vi "GetMatlabTempParamData.vi"(10 "index":dbl, 11 "ExpID":string) -> (3 "Matlab param data":T1[](array[typedef]))   [LabVIEW 2017]
uses:
  Types/MatlabDataBundle.ctl
  Types/MatlabDataType.ctl
panel:
  out "Param Data before convert":T1[](array[typedef])
  in  "Clear Temp?":bool=TRUE
  out "error out":errorcluster
  in  "error in":errorcluster
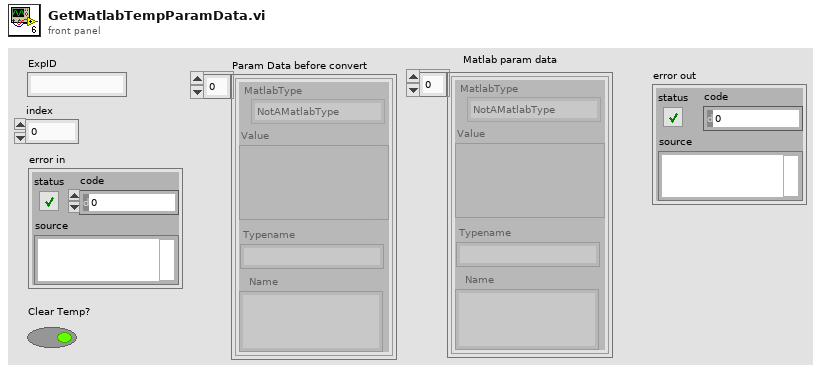
[diagram p1: front panel]
types:
  T1 = typedef "MatlabDataBundle.ctl" = cluster{"MatlabType":T2, "Value":variant, "Name":string, "Typename":string}
  T2 = typedef "MatlabDataType.ctl" = enum16{"NotAMatlabType", "Real", "Complex", "String", "Boolean"}
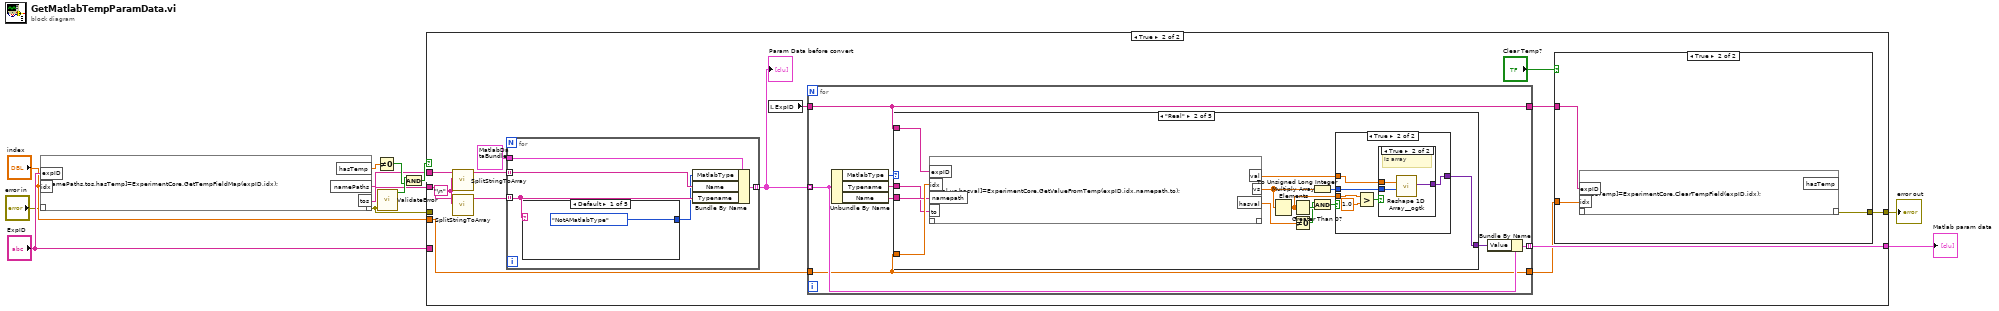
[diagram p0: block diagram]
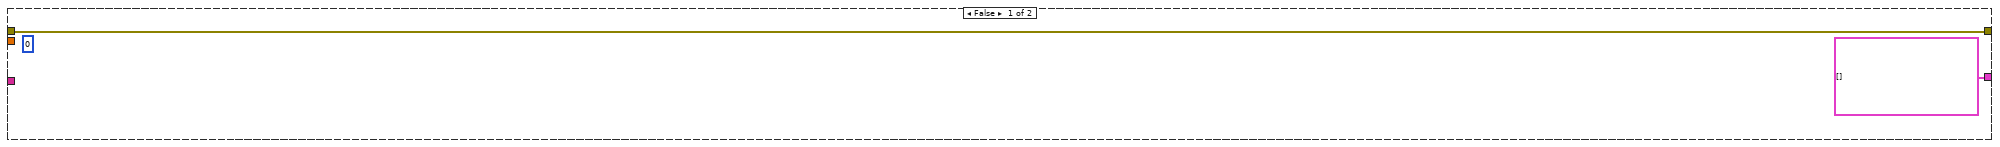
[diagram p2: hidden frame]
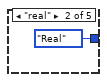
[diagram p3: hidden frame]
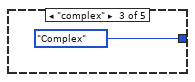
[diagram p4: hidden frame]
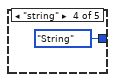
[diagram p5: hidden frame]
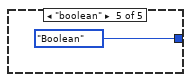
[diagram p6: hidden frame]
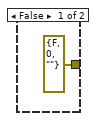
[diagram p7: hidden frame]
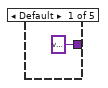
[diagram p8: hidden frame]
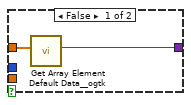
[diagram p9: hidden frame]
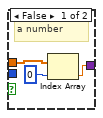
[diagram p10: hidden frame]
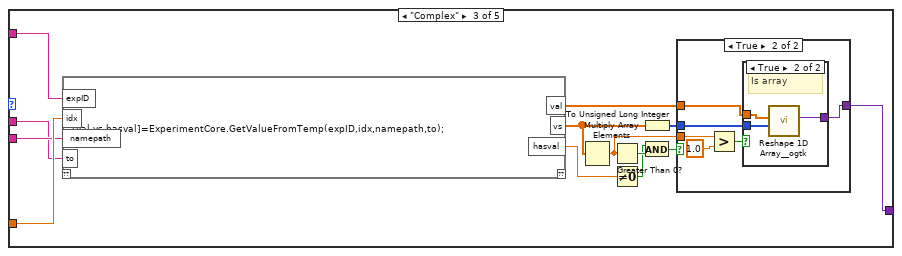
[diagram p11: hidden frame]
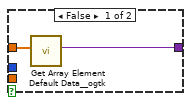
[diagram p12: hidden frame]
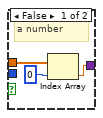
[diagram p13: hidden frame]
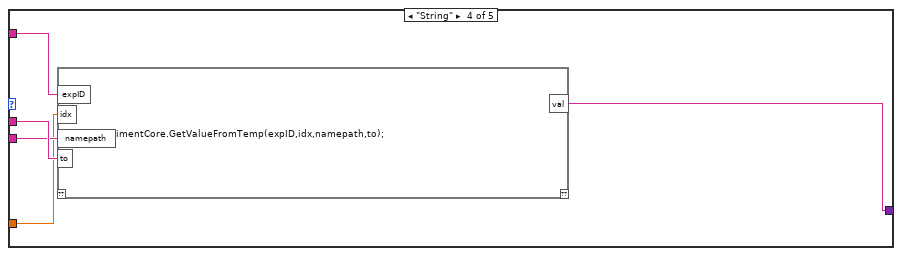
[diagram p14: hidden frame]
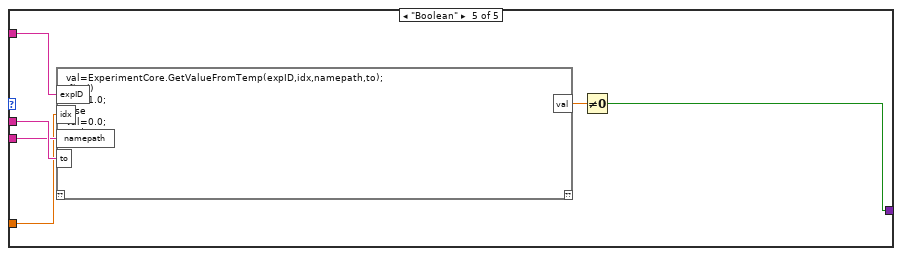
[diagram p15: hidden frame]
diagram:
  n1 = script code="[namePaths,tos,hasTemp]=ExperimentCore.GetTempFieldMap(expID,idx);"("??"="error in", "expID"="ExpID", "idx"="index") -> ("??"=w8:errorcluster, "hasTemp"=w11:dbl, "namePaths"=w1:string, "tos"=w2:string)
  n2 = Not Equal To 0?(x=w11) -> (x != 0?=w6:bool)
  n3 = call "ValidateError.vi"("error in (no error)"=w8) -> ("NoError?"=w7:bool)  [unwired: 9 in, 1 out]
  n4 = And(x=w7, y=w6) -> (x .and. y?=w5:bool)
  n5 = case shown="True" w5 {
    tunnel: [T1[] [] w28] -> w12
    tunnel: "ExpID" -> [_ _]
    tunnel: "index" -> [_ w27]
    tunnel: w8 -> [w13 _]
    tunnel: [w13 w16] -> w3
    tunnel: w2 -> [_ w21]
    tunnel: w1 -> [_ w20]
    frame False {
      (unwired) 0
    }
    frame True {
      w22 = "\n"
      n6 = call "SplitStringToArray.vi"("search string/char (-)"=w22, "String in"=w20) -> ("Split(s)"=w24:string[])  [unwired: 9 in]
      n7 = call "SplitStringToArray.vi"("search string/char (-)"=w22, "String in"=w21) -> ("Split(s)"=w25:string[])  [unwired: 9 in]
      n8 = for {
        tunnel: w24 -> [w32] mode=indexing
        tunnel: w25 -> [w30] mode=indexing
        tunnel: T1 {"MatlabType"=enum."NotAMatlabType", "Value"=variant, "Name"="", "Typename"=""} ("MatlabDataBundle") -> [w33]
        tunnel: [w31] -> w19 mode=indexing
        n9 = case shown="Default" w30 {
          tunnel: [MatlabDataType."NotAMatlabType" ("MatlabType") MatlabDataType."Real" ("MatlabType") MatlabDataType."Complex" ("MatlabType") MatlabDataType."String" ("MatlabType") MatlabDataType."Boolean" ("MatlabType")] -> w29
          frame Default {
          }
          frame "real" {
          }
          frame "complex" {
          }
          frame "string" {
          }
          frame "boolean" {
          }
        }
        n10 = Bundle By Name(cluster=w33, "MatlabType"=w29, "Name"=w32, "Typename"=w30) -> (w31:T1)
      }
      "Param Data before convert" <- w19
      n11 = local read "ExpID"() -> (w18:string)
      n12 = for {
        tunnel: w19 -> [w47] mode=indexing
        tunnel: [w46] -> w28 mode=indexing
        tunnel: w27 -> [w43]
        tunnel: w18 -> [w44]
        tunnel: [w44] -> w17
        tunnel: [w43] -> w15
        n13 = Unbundle By Name(w47) -> ("MatlabType"=w45:T2, "Typename"=w50:string, "Name"=w49:string)
        n14 = case shown="\"Real\"" w45 {
          tunnel: [variant ("Reshaped VArray") w58 w85 w110 w115] -> w48
          tunnel: w44 -> [_ w64 w91 w109 w114]
          tunnel: w50 -> [_ w61 w88 w108 w113]
          tunnel: w49 -> [_ w62 w89 w107 w112]
          tunnel: w43 -> [_ w63 w90 w106 w111]
          frame Default {
          }
          frame "Real" {
            n15 = script code="[val,vs,hasval]=ExperimentCore.GetValueFromTemp(expID,idx,namepath,to);"("expID"=w64, "idx"=w63, "to"=w61, "namepath"=w62) -> ("val"=w59:dbl[], "vs"=w56:dbl[], "hasval"=w57:dbl)  [unwired: 1 in, 1 out]
            n16 = Multiply Array Elements(1:w56) -> (0:w54:dbl)
            n17 = Greater Than 0?(x=w54) -> (x > 0?=w55:bool)
            n18 = Not Equal To 0?(x=w57) -> (x != 0?=w53:bool)
            n19 = To Unsigned Long Integer(number=w56) -> (unsigned 32bit integer=w60:u32[])
            n20 = And(x=w53, y=w55) -> (x .and. y?=w52:bool)
            n21 = case shown="True" w52 {
              tunnel: w60 -> [_ w68]
              tunnel: w59 -> [w66 w69]
              tunnel: [w65 w67] -> w58
              tunnel: w54 -> [_ w71]
              frame False {
                n22 = call <userlib>:"Get Array Element Default Data__ogtk.vi"("Array"=w66) -> ("Array Element Default Data"=w65:variant)  [unwired: 9 in, 1 out]
              }
              frame True {
                n23 = Greater?(x=w71, y=1.0 ("x")) -> (0:w70:bool)
                n24 = case shown="True" w70 {
                  tunnel: w69 -> [w75 w78]
                  tunnel: w68 -> [_ w77]
                  tunnel: [w74 w76] -> w67
                  frame False {
                    # "a number"
                    n25 = Index Array(array=w75, index=0) -> (element=w74:dbl)
                  }
                  frame True {
                    # "Is array"
                    n26 = call <userlib>:"Reshape 1D Array__ogtk.vi"("Size(s)"=w77, "1D Array"=w78) -> ("Reshaped VArray"=w76:variant)  [unwired: 8 in, 1 out]
                  }
                }
              }
            }
          }
          frame "Complex" {
            n27 = script code="[val,vs,hasval]=ExperimentCore.GetValueFromTemp(expID,idx,namepath,to);"("expID"=w91, "idx"=w90, "to"=w88, "namepath"=w89) -> ("val"=w86:cdb[], "vs"=w83:dbl[], "hasval"=w84:dbl)  [unwired: 1 in, 1 out]
            n28 = Multiply Array Elements(1:w83) -> (0:w81:dbl)
            n29 = Greater Than 0?(x=w81) -> (x > 0?=w82:bool)
            n30 = Not Equal To 0?(x=w84) -> (x != 0?=w80:bool)
            n31 = To Unsigned Long Integer(number=w83) -> (unsigned 32bit integer=w87:u32[])
            n32 = And(x=w80, y=w82) -> (x .and. y?=w79:bool)
            n33 = case shown="True" w79 {
              tunnel: w87 -> [_ w95]
              tunnel: w86 -> [w93 w96]
              tunnel: [w92 w94] -> w85
              tunnel: w81 -> [_ w98]
              frame False {
                n34 = call <userlib>:"Get Array Element Default Data__ogtk.vi"("Array"=w93) -> ("Array Element Default Data"=w92:variant)  [unwired: 9 in, 1 out]
              }
              frame True {
                n35 = Greater?(x=w98, y=1.0 ("x")) -> (0:w97:bool)
                n36 = case shown="True" w97 {
                  tunnel: w96 -> [w102 w105]
                  tunnel: w95 -> [_ w104]
                  tunnel: [w101 w103] -> w94
                  frame False {
                    # "a number"
                    n37 = Index Array(array=w102, index=0) -> (element=w101:cdb)
                  }
                  frame True {
                    # "Is array"
                    n38 = call <userlib>:"Reshape 1D Array__ogtk.vi"("Size(s)"=w104, "1D Array"=w105) -> ("Reshaped VArray"=w103:variant)  [unwired: 8 in, 1 out]
                  }
                }
              }
            }
          }
          frame "String" {
            n39 = script code="val=ExperimentCore.GetValueFromTemp(expID,idx,namepath,to);"("expID"=w109, "idx"=w106, "namepath"=w107, "to"=w108) -> ("val"=w110:string)  [unwired: 1 in, 1 out]
          }
          frame "Boolean" {
            n40 = script code="val=ExperimentCore.GetValueFromTemp(expID,idx,namepath,to);\nif(val)\nval=1.0;\nelse\nval=0.0;\nend"("expID"=w114, "idx"=w111, "namepath"=w112, "to"=w113) -> ("val"=w116:dbl)  [unwired: 1 in, 1 out]
            n41 = Not Equal To 0?(x=w116) -> (x != 0?=w115:bool)
          }
        }
        n42 = Bundle By Name(cluster=w47, "Value"=w48) -> (w46:T1)
      }
      n43 = case shown="True" "Clear Temp?" {
        tunnel: w17 -> [_ w42]
        tunnel: w15 -> [_ w41]
        tunnel: [errorcluster {"status"=FALSE, "code"=0, "source"=""} ("error IO") w40] -> w16
        frame False {
        }
        frame True {
          n44 = script code="[hasTemp]=ExperimentCore.ClearTempField(expID,idx);"("expID"=w42, "idx"=w41) -> ("??"=w40:errorcluster)  [unwired: 1 in, 1 out]
        }
      }
    }
  }
  "Matlab param data" <- w12
  "error out" <- w3
